vi "Init wave memory.vi"() -> ()   [LabVIEW 2014]
uses:
  <vilib>/Utility/file.llb/Read From Spreadsheet File (I64).vi
panel:
  out "Text file path":path
  out "Init Data Out":i64[](array[numeric])
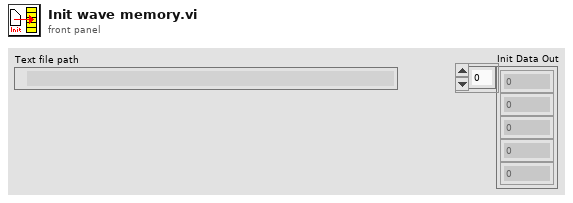
[diagram p1: front panel]
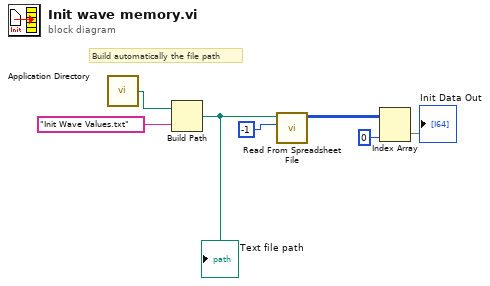
[diagram p0: block diagram]
diagram:
  # "Build automatically the file path"
  n1 = call <vilib>:"Application Directory.vi"() -> ("Application Directory"=w3:path)
  n2 = Build Path(base path=w3, name or relative path="Init Wave Values.txt") -> (appended path=w1:path)
  "Text file path" <- w1
  n3 = call-poly <vilib>:"Read From Spreadsheet File.vi"("number of rows (all:-1)"=-1, "file path (dialog if empty)"=w1) -> ("all rows"=w6:i64[][])  [unwired: 5 in, 4 out]
  n4 = Index Array(array=w6, index (col)=0 ("disabled index (col)")) -> (element=→"Init Data Out":i64[])  [unwired: 1 in]
